vi "PvgeneratorOP300.vi"(8 "errin":errorcluster, 10 "network":path, 11 "path in":path) -> (0 "sortie d'erreur":errorcluster caption="errout", 1 "network out":path, 2 "tout bon":bool, 3 "Chaîne":string)   [LabVIEW 2020]
uses:
  SubVI/CheminDeBase.vi
  VG/IS30%.vi
  VG/PN.vi
  <vilib>/Utility/config.llb/NI_LVConfig.lvlib
panel:
  out "nombre de remplacements":i32
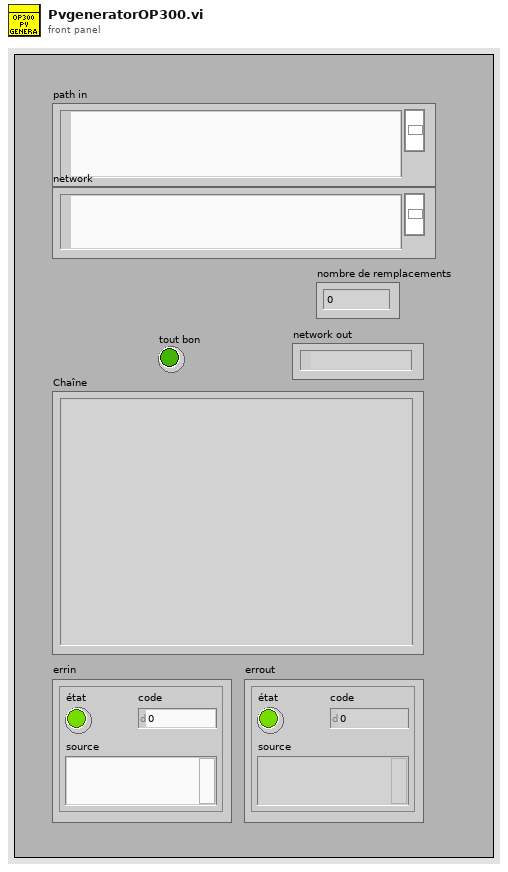
[diagram p1: front panel]
types:
  T1 = enum16{"open", "replace", "create", "open or create", "replace or create", "replace or create with confirmation"}
  T2 = typedef "NI_LVConfig.lvlib/Config Data RefNum.ctl" = refnum<k1>
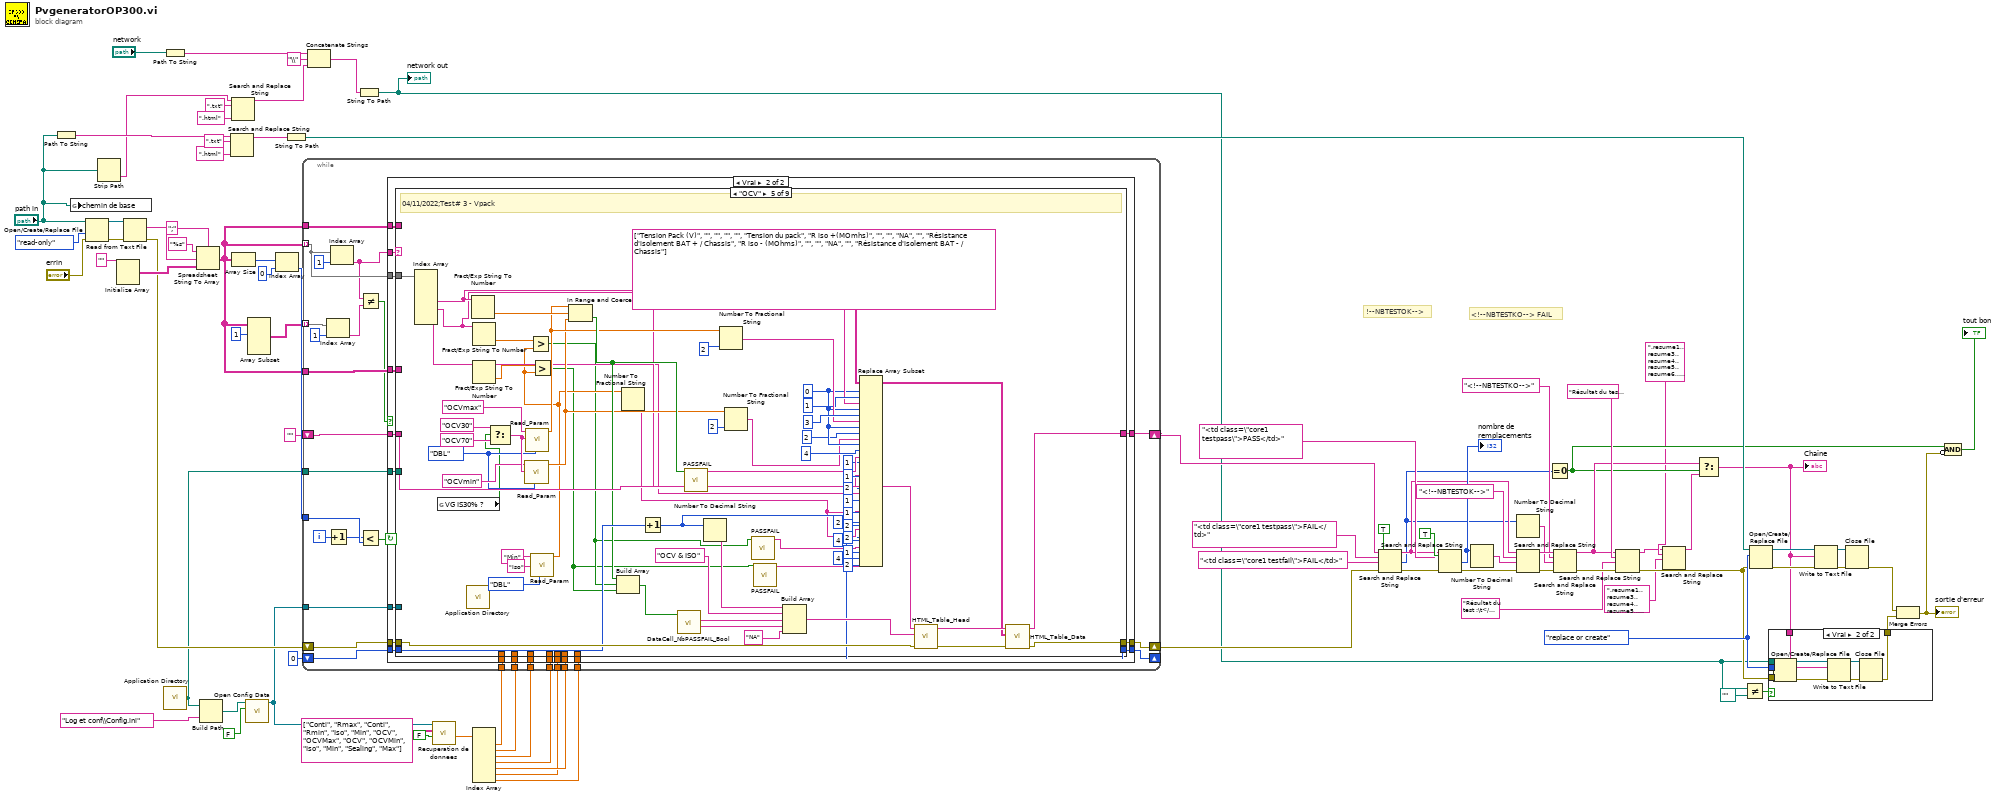
[diagram p0: block diagram]
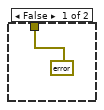
[diagram p2: hidden frame]
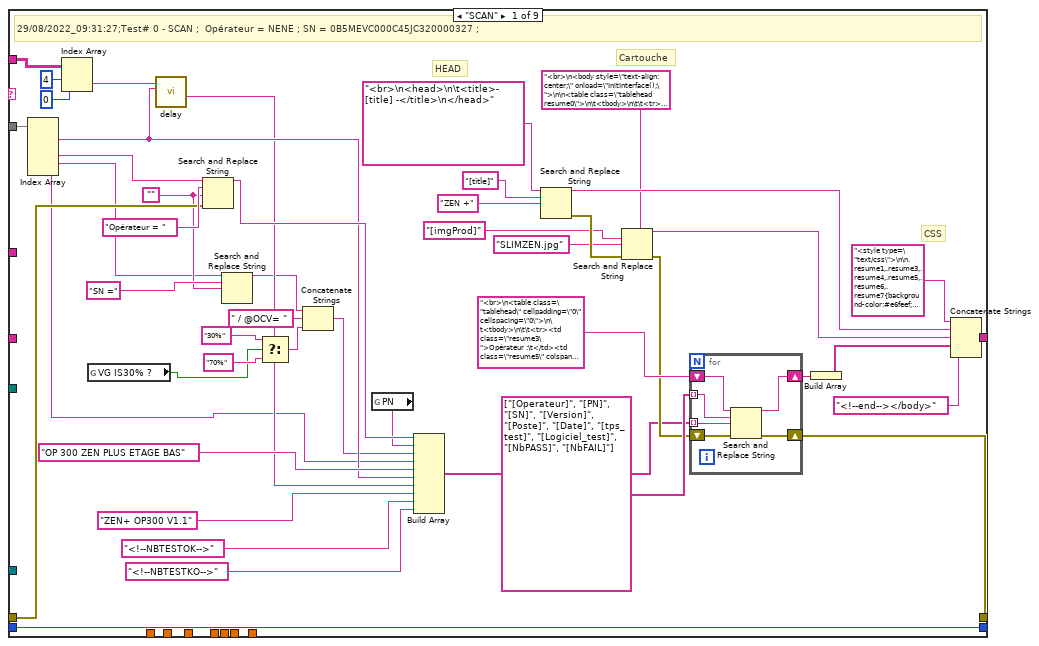
[diagram p4: hidden frame]
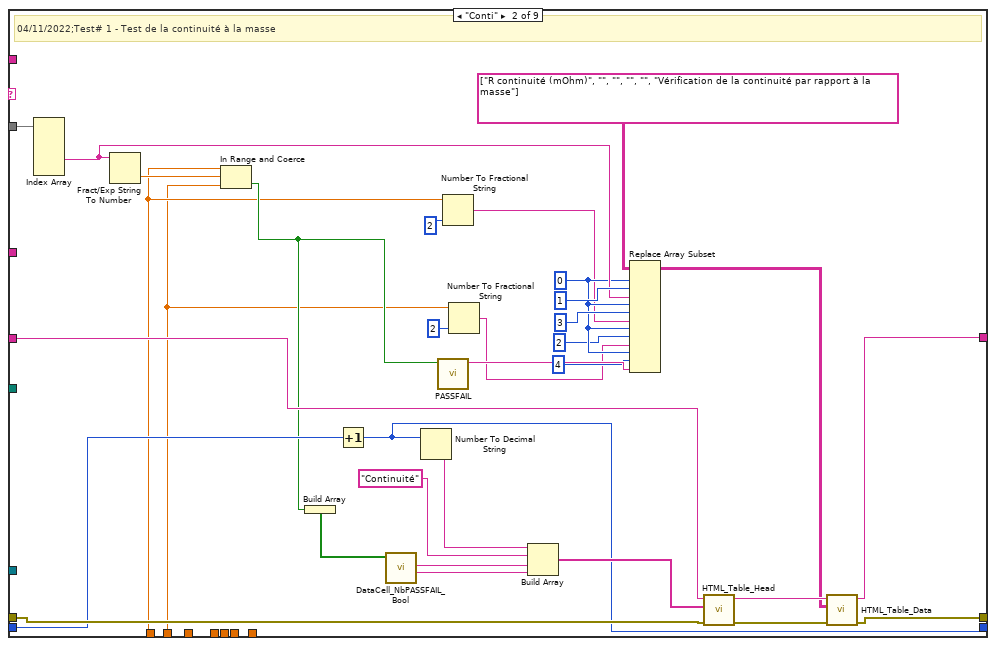
[diagram p5: hidden frame]
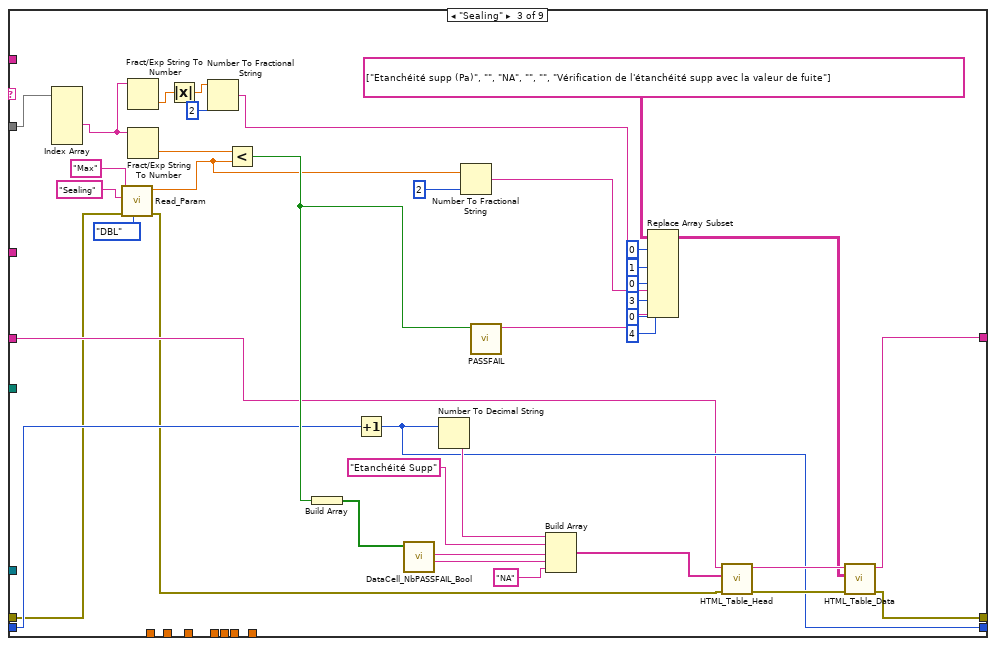
[diagram p6: hidden frame]
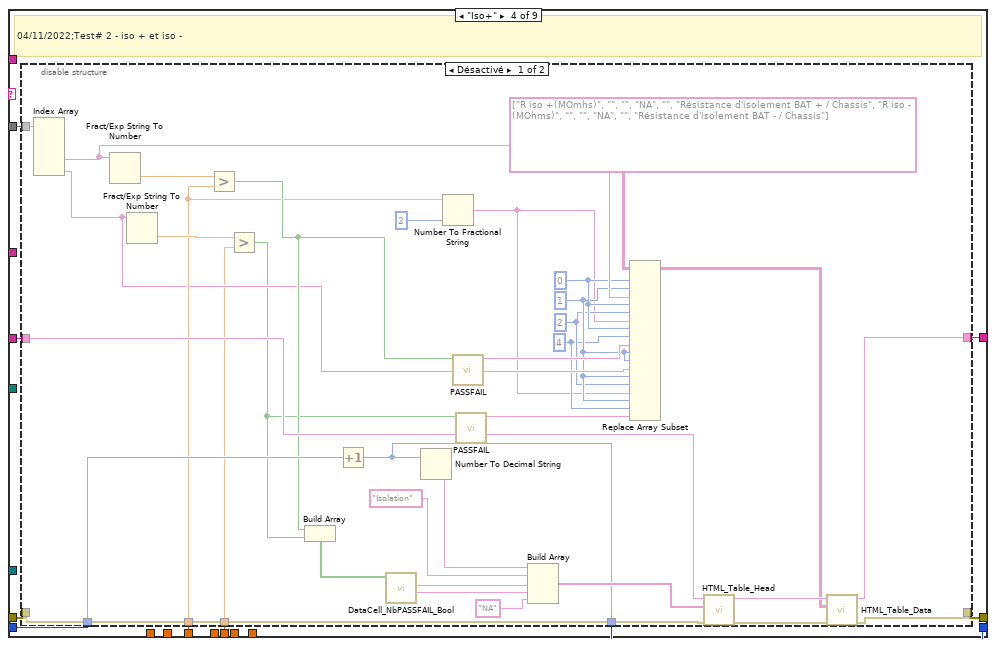
[diagram p7: hidden frame]
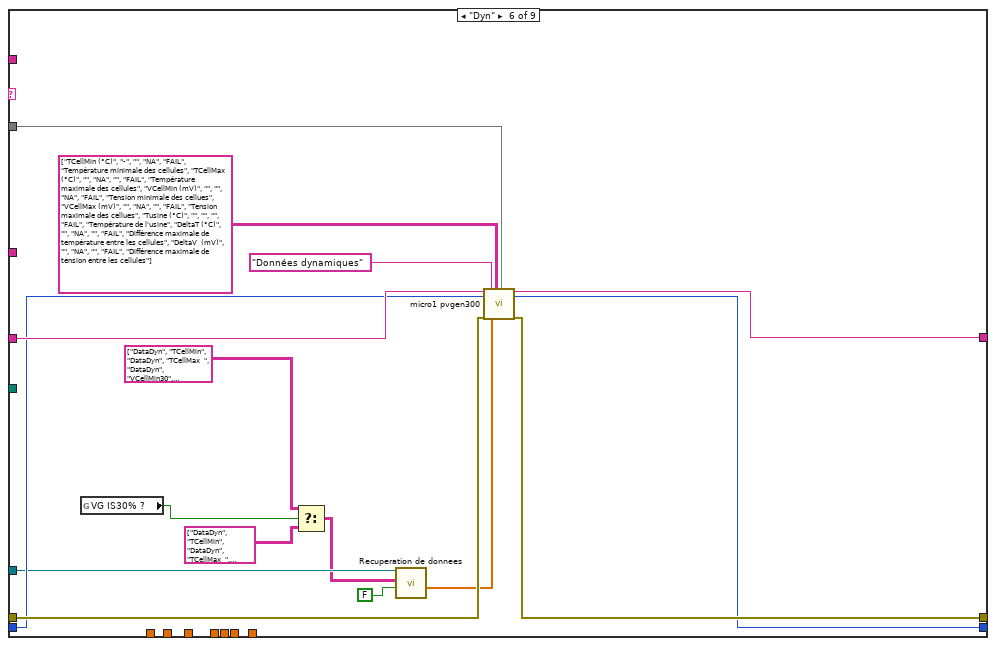
[diagram p9: hidden frame]
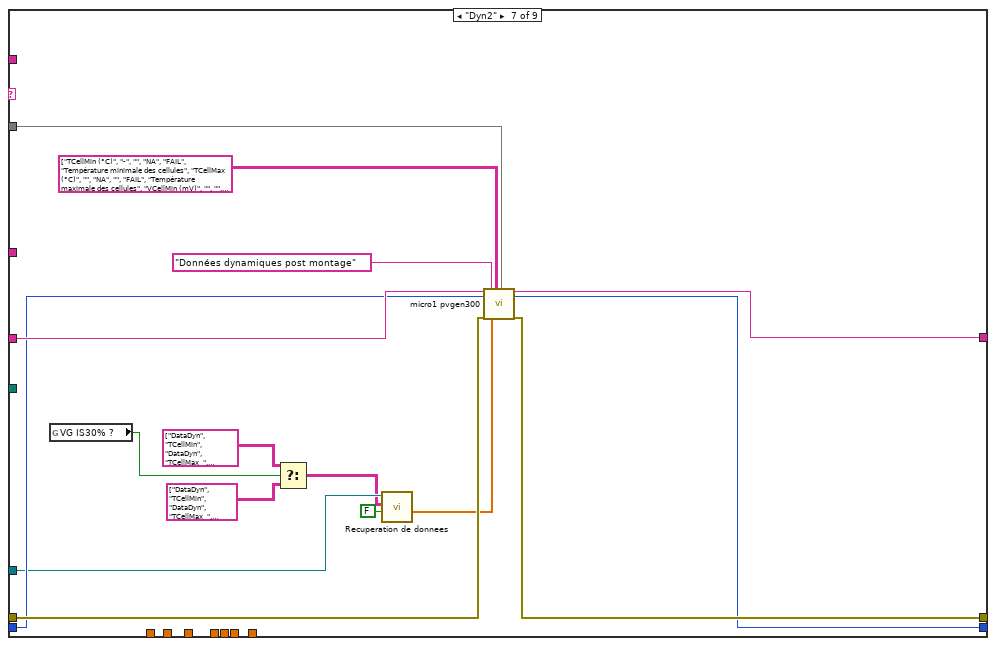
[diagram p10: hidden frame]
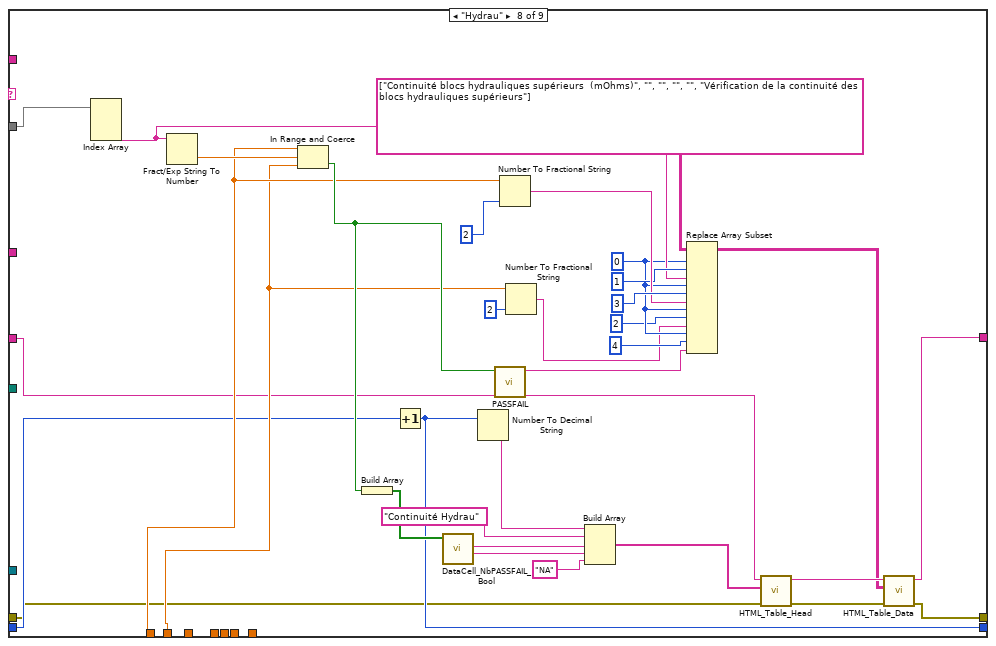
[diagram p11: hidden frame]
diagram:
  w47 = T1."replace or create" ("opération (0 : open)")
  # "<!--NBTESTKO--> FAIL"
  # "!--NBTESTOK-->"
  n1 = Path To String(path="path in") -> (string=w69:string)
  n2 = global write "CheminDeBase.vi" "chemin de base"("path in") -> ()
  n3 = Open/Create/Replace File(file path (use dialog)="path in", error in="errin", access (0:read/write)=enum16{"read/write", "read-only", "write-only"}."read-only" ("accès (0 : read/write)")) -> (refnum out=w70:refnum<file>, error out=w87:errorcluster)  [unwired: 3 in, 1 out]
  n4 = Strip Path(path="path in") -> (name=w29:string)  [unwired: 1 out]
  n5 = Initialize Array("") -> (w85:string[][])  [unwired: 2 in]
  n6 = Read from Text File(file (use dialog)=w70, error in=w87) -> (text=w83:string, error out=w75:errorcluster)  [unwired: 2 in, 2 out]
  n7 = Path To String(path="network") -> (string=w28:string)
  n8 = call <vilib>:"Application Directory.vi"() -> ("Application Directory"=w2:path)
  n9 = Spreadsheet String To Array(delimiter (Tab)=";" ("séparateur (Tabulation)"), format string="%s" ("chaîne de format"), spreadsheet string=w83, array type (2D Dbl)=w85) -> (array=w8:string[][])
  n10 = Build Path(base path=w2, name or relative path="Log et conf\\Config.ini") -> (appended path=w23:path)
  n11 = Search and Replace String(input string=w69, search string=".txt" ("chaîne recherchée"), replace string=".html" ("chaîne de remplacement (\"\")")) -> (result string=w66:string)  [unwired: 5 in, 3 out]
  n12 = Search and Replace String(input string=w29, search string=".txt" ("chaîne recherchée"), replace string=".html" ("chaîne de remplacement (\"\")")) -> (result string=w26:string)  [unwired: 5 in, 3 out]
  n13 = Array Size(array=w8) -> (size(s)=w81:i32[])
  n14 = call <vilib>:"Open Config Data.vi"("create file if necessary (T)"=FALSE, "configuration file path"=w23) -> ("refnum"=w3:T2)  [unwired: 7 in, 2 out]
  n15 = Array Subset(array=w8, index (row)=1 ("indice")) -> (w6:string[][])  [unwired: 3 in]
  n16 = Index Array(array=w81, index=0 ("indice")) -> (element=w79:i32)
  n17 = String To Path(string=w66) -> (path=w65:path)
  n18 = Concatenate Strings(w28, "\\" ("chaîne"), w26) -> (w25:string)
  n19 = String To Path(string=w25) -> (path=w30:path)
  "network out" <- w30
  n20 = call "Recuperation de donnees.vi"("Est-ce un string?"=FALSE, "Array in"=string[][] [["Conti", "Rmax"], ["Conti", "Rmin"], ["Iso", "Min"], ["OCV", "OCVMax"], ["OCV", "OCVMin"], ["Iso", "Min"], ["Sealing", "Max"]], "Refnum in"=w3) -> ("Array"=w18:dbl[])  [unwired: 7 in, 1 out]
  n21 = Index Array(array=w18) -> (element #1=w17:dbl, element #2=w16:dbl, element #3=w15:dbl, element #4=w14:dbl, element #5=w13:dbl, element #6=w5:dbl, element #7=w4:dbl)  [unwired: 7 in]
  n22 = while {
    tunnel: w79 -> [w115]
    tunnel: w8 -> [w112] mode=indexing
    shift-right: [w111] -> w62
    shift-left: w75 -> [w110]
    shift-right: [w104] -> w64
    shift-left: "" -> [w109]
    shift-right: [w107] -> _
    shift-left: 0 -> [w108]
    tunnel: w8 -> [w106]
    tunnel: w17 -> [w103]
    tunnel: w16 -> [w102]
    tunnel: w8 -> [w101]
    tunnel: w15 -> [w100]
    tunnel: w14 -> [w99]
    tunnel: w13 -> [w98]
    tunnel: w6 -> [w96] mode=indexing
    tunnel: w5 -> [w92]
    tunnel: w4 -> [w91]
    tunnel: w3 -> [w90]
    tunnel: w2 -> [w89]
    i -> [w116]
    stop <- w114 continue-if-true
    n23 = Index Array(array=w96, index=1 ("indice")) -> (element=w95:string)
    n24 = Increment(x=w116) -> (x+1=w105:i32)
    n25 = Index Array(array=w112, index=1 ("indice")) -> (element=w94:string)
    n26 = Less?(x=w105, y=w115) -> (x < y?=w114:bool)
    n27 = Not Equal?(x=w94, y=w95) -> (x != y?=w93:bool)
    n28 = case shown="Vrai" w93 {
      tunnel: w112 -> [_ w138]
      tunnel: [w118 w137] -> w111
      tunnel: w110 -> [w118 w136]
      tunnel: w109 -> [w119 w135]
      tunnel: w108 -> [w117 w134]
      tunnel: [w117 w133] -> w107
      tunnel: w106 -> [_ w132]
      tunnel: [w119 w131] -> w104
      tunnel: w94 -> [_ w130]
      tunnel: w103 -> [_ w120]
      tunnel: w102 -> [_ w129]
      tunnel: w101 -> [_ w128]
      tunnel: w100 -> [_ w127]
      tunnel: w99 -> [_ w126]
      tunnel: w98 -> [_ w125]
      tunnel: w92 -> [_ w124]
      tunnel: w91 -> [_ w123]
      tunnel: w90 -> [_ w122]
      tunnel: w89 -> [_ w121]
      frame False {
      }
      frame True {
        n29 = case shown="\"OCV\"" w130 {
          tunnel: w136 -> [w183 w216 w231 w270 w362 w386 w402 w405 w438]
          tunnel: w138 -> [w185 w217 w246 w271 w363 w383 w399 w411 _]
          tunnel: [w162 w215 w235 w269 w361 w385 w401 w406 w438] -> w137
          tunnel: w135 -> [_ w214 w232 w268 w360 w382 w398 w404 w436]
          tunnel: w134 -> [w161 w213 w234 w267 w359 w381 w397 w408 w437]
          tunnel: [w161 w212 w233 w266 w358 w380 w396 w407 w437] -> w133
          tunnel: w132 -> [_ _ _ _ _ _ _ _ _]
          tunnel: [w160 w211 w236 w265 w357 w384 w400 w403 w436] -> w131
          tunnel: w129 -> [_ w194 _ _ _ _ _ w409 _]
          tunnel: w128 -> [w154 _ _ _ _ _ _ _ _]
          tunnel: w127 -> [_ _ _ w264 _ _ _ _ _]
          tunnel: w126 -> [_ _ _ _ _ _ _ _ _]
          tunnel: w125 -> [_ _ _ _ _ _ _ _ _]
          tunnel: w124 -> [_ _ _ w263 _ _ _ _ _]
          tunnel: w123 -> [_ _ _ _ _ _ _ _ _]
          tunnel: w122 -> [_ _ _ _ _ w379 w395 _ _]
          tunnel: w121 -> [_ _ _ _ _ _ _ _ _]
          tunnel: w120 -> [_ w195 _ _ _ _ _ w410 _]
          frame "SCAN" {
            w156 = ""
            # "Cartouche"
            # "HEAD"
            # "CSS"
            # "29/08/2022_09:31:27;Test# 0 - SCAN ;  Opérateur = NENE ; SN = 0B5MEVC000C45JC320000327 ;"
            n30 = Index Array(array=w185) -> (element #1=w150:string, element #3=w159:string, element #4=w155:string, element #5=w139:string)  [unwired: 5 in, 1 out]
            n31 = Index Array(array=w154, index (row)=4, index (col)=0 ("disabled index (col)")) -> (element=w151:string)
            n32 = global read "IS30%.vi" "VG IS30% ?"() -> (w141:bool)
            n33 = call "delay.vi"("String"=w150, "String 2"=w151) -> ("Delay calculé"=w149:string)  [unwired: 9 in]
            n34 = Search and Replace String(input string=w159, search string="Opérateur = " ("chaîne recherchée"), replace string=w156, error in=w183) -> (result string=w158:string)  [unwired: 4 in, 3 out]
            n35 = Search and Replace String(input string=w155, search string="SN =" ("chaîne recherchée"), replace string=w156) -> (result string=w147:string)  [unwired: 5 in, 3 out]
            n36 = Select(t="30%" ("y"), s=w141, f="70%" ("y")) -> (s? t:f=w144:string)
            n37 = Concatenate Strings(w147, " / @OCV= " ("chaîne"), w144) -> (w146:string)
            n38 = global read "PN.vi" "PN"() -> (w140:string)
            n39 = Build Array(w158, w140, w146, w139, "OP 300 ZEN PLUS ETAGE BAS" ("chaîne"), w150, w149, "ZEN+ OP300 V1.1" ("chaîne"), "<!--NBTESTOK-->" ("chaîne"), "<!--NBTESTKO-->" ("chaîne")) -> (w163:string[])
            n40 = Search and Replace String(input string="<br>\n<head>\n\t<title>- [title] -</title>\n</head>", search string="[title]" ("chaîne recherchée"), replace string="ZEN +" ("Title")) -> (result string=w179:string, error out=w178:errorcluster)  [unwired: 5 in, 2 out]
            n41 = Search and Replace String(input string="<br>\n<body style=\"text-align: center;\" onload=\"InitInterface();\">\n\n<table class=\"tablehead resume0\">\n\t<tbody>\n\t\t<tr>\n\t\t\t<td> <img src=\"[imgProd]\" style=\"width:194px;height:100px\" class=\"left\"></td>\n\t\t\t<td> <div class=\"center\">PROCES VERBAL DE TEST AUTOMATIQUE</div><div class=\"center\">Zen Plus OP 300</div><br class=\"center\"><div class=\"center\">Forseepower</div></td>\n\t\t\t<td> <img src=\"LOGO FORSEE.png\" style=\"width:194px;height:100px\"  class=\"right\"></td>\n\t\t</tr>\n\t</tbody>\n</table>", search string="[imgProd]", replace string="SLIMZEN.jpg" ("imgProd"), error in=w178) -> (result string=w176:string, error out=w173:errorcluster)  [unwired: 4 in, 2 out]
            n42 = for {
              shift-right: [w190] -> w172
              shift-left: "<br>\n<table class=\"tablehead\" cellpadding=\"0\" cellspacing=\"0\">\n\t<tbody>\n\t\t<tr><td class=\"resume3\">Opérateur :\t</td><td class=\"resume5\" colspan=\"3\">[Operateur]</td></tr>\n\t\t<tr><td class=\"resume3\">PN : </td><td class=\"resume5\" colspan=\"3\">[PN]</td></tr>\n\t\t<tr><td class=\"resume3\">SN : </td><td class=\"resume5\" colspan=\"3\">[SN]</td></tr>\n\t\t<tr><td class=\"resume3\">Version : </td><td class=\"resume5\" colspan=\"3\">[Version]</td></tr>\n\t\t<tr><td class=\"resume3\">Poste : </td><td class=\"resume5\" colspan=\"3\">[Poste]</td></tr>\t\t\n\t\t<tr><td class=\"resume3\">Date du test : </td><td class=\"resume5\" colspan=\"3\">[Date]</td></tr>\n\t\t<tr><td class=\"resume3\">Temps de test : </td><td class=\"resume5\" colspan=\"3\">[tps_test]</td></tr>\n\t\t<tr><td class=\"resume3\">Logiciel de test :\t</td><td class=\"resume5\" colspan=\"3\">[Logiciel_test]</td></tr>\n\t\t<tr><td class=\"resume3\">Résultat du test :\t</td><td class=\"resume5\" colspan=\"3\"><div><span style=\"float:left\" id=\"result\"><font size = \"5pt\" color=\"green\"><b>CONFORME</b></font><b><font size = \"5pt\"> ( </font><font size = \"5pt\" color=\"green\">[NbPASS] PASS </font>  <font size = \"5pt\"> / </font><font size = \"5pt\" color=\"red\">[NbFAIL] FAIL</font> <font size = \"5pt\"> ) </font></b></span></div></td></tr>\n\t</tbody>\n</table>" -> [w191]
              tunnel: string[] ["[Operateur]", "[PN]", "[SN]", "[Version]", "[Poste]", "[Date]", "[tps_test]", "[Logiciel_test]", "[NbPASS]", "[NbFAIL]"] -> [w187] mode=indexing
              tunnel: w163 -> [w186] mode=indexing
              shift-right: [w188] -> w162
              shift-left: w173 -> [w189]
              n43 = Search and Replace String(input string=w191, search string=w187, replace string=w186, error in=w189) -> (result string=w190:string, error out=w188:errorcluster)  [unwired: 4 in, 2 out]
            }
            n44 = Build Array(w172) -> (w171:string[])
            n45 = Concatenate Strings("<style type=\"text/css\">\n\n.resume1,.resume3,.resume4,.resume5,.resume6,.resume7{background-color:#e6feef;padding:7px;border:1px solid black;}\n.resume0{border:1px solid black;background-color:#e6feef;font-weight: bold;padding:0px;text-align: center;}\n.resume1{width:350px;text-align:right;font-weight:bold;}\n.resume3{width:350px;text-align:right;border-top:0px solid black;font-weight:bold;}\n.resume4{border-left:0px solid black;width:290px;}\n.resume5{width:290px;border-left:0px solid black;border-top:0px solid black;}\n.resume6{border-left:0px solid black;width:60px;}\n.resume7{border-left:0px solid black;border-top:0px solid black;width:60px;}\n.title1{text-align: left;background-color:#e6f4fe;padding:10px;border:1px solid #101010;}\n.title2{width: 30px;text-align: center;background-color:#e6f4fe;padding:1px;border:1px solid #101010;border-left:0px solid black;font-weight: bold;}\n.title2 a:link{text-decoration:none;}\n.entete0,.entete1,.entete2,.time2{text-align: center;background-color:#feeec9;padding:7px;border:1px solid black;font-weight: bold;}\n.entete0{width:45px;border-right:0px solid black;}\n.entete1{width:505px;}\n.entete2{width:95px;border-right:0px solid black;}\n.time2{border-left:0px solid black;width:145px;font-size:11px;}\n.core0,.core1,.core2,.core3,.core4,.time{text-align: center;background-color:#fafed3;padding:7px;border:1px solid black;}\n.core0, .core1,.core3,.core4{width:95px;border-top:0px solid black;border-right:0px solid black;}\n.core0{width:45px;}\n.core2{border-top:0px solid black;width:505px;}\n.core3{width:200px;}\n.core4{width:300px;}\n.time{width:145px;border-top:0px solid black;border-left:0px solid black;font-size:11px;}\n.false .core0,.false .core1,.false .core2,.false .core3,.false .core4,.false .time{background-color:#f4f4f4;}\n.false .entete0,.false .entete1,.false .entete2,.false .time2{background-color:#dadada;}\n.false .title1,.false .title2,.false .resultentete .testpass,.false .resultentete .testfail,.false .resultentete .testtime{background-color:#c5cac9;color: blue;}\n.false .title2 a:link{text-decoration:none;color: blue;}\n.comment1,.comment2,.time3{width: 890px;background-color:#e9e8e9;padding:7px;border:1px solid black;border-top:0px solid black;text-align:left;}\n.comment2{border-right:0px solid black;width: 45px;text-align: center;}\n.time3{width: 145px;border-left:0px solid black;font-size:11px;}\n.fixe1{background: -moz-linear-gradient(center top , #101010 10%, #555555 80%) repeat scroll 0 0 transparent;background: -webkit-gradient(linear, left top, left bottom, from(#101010), to(#555555));border:2px solid orange;position : fixed;margin-top:20px;display:none;overflow-y:scroll;max-height:350px;text-shadow: 0px 0px 0 #333333;text-align:left;font-size:10px;padding:10px;margin-left:-162px;border-radius: 15px 15px 15px 15px;}\n.menufixe, .menufixelock{background: -moz-linear-gradient(center top , #101010 80%, transparent 20%) repeat scroll 0 0 transparent;background: -webkit-gradient(linear, left top, left bottom, from(#101010), color-stop(0.65, #101010), to(transparent)) repeat scroll 0 0 transparent;margin: -52px 0px 0px -9px;width:100%;position:fixed;height:55px;-moz-transition: margin 1s;-webkit-transition: margin 1s;}\n.menufixelock, .menufixe:hover{margin: -9px 0px 0px -9px;}\n.lockmenu, .separation,.separationmenu{text-align:center;background: -moz-linear-gradient(center top , #555555 10%, #111111 80%) repeat scroll 0 0 transparent;background: -webkit-gradient(linear, left top, left bottom, from(#555555), to(#111111));border: 1px solid white;border-radius: 10px 10px 10px 10px;box-shadow: 0 -1px 1px #555555 inset;color: #999999;font-weight: bold;width: 100px;padding: 2px;text-decoration: none;}\n.tablehead{width: 1000px;font-family: Verdana;font-size: 12px;margin-left: auto;margin-right: auto;}\n.tablenull{font-family: Verdana;font-size: 11px;margin-left: auto;margin-right: auto;}\n.separationmenu:hover div{display: inline;}\n.lockmenu:hover, .separation:hover,.separationmenu:hover{border: 1px solid orange;cursor:pointer;}\n.lockmenu:hover{border: 1px solid red;cursor:pointer;}\n.separationright{padding:10px;}\ndiv a:link{text-decoration:none;color:#cbcbcb;}\ndiv a:hover{text-decoration:underline;color:#cbcbcb;}\nspan a:link{text-decoration:none;color:#cbcbcb;}\nspan a:hover{text-decoration:none;color:#cbcbcb;}\n.false{color: blue;}\n.testpass{color: green;font-weight: bold;}\n.testfail{color: red;font-weight: bold;}\n.testtime{color: blue;font-weight: bold;}\n.resultentete{font-weight: bold;font-size: 11px;min-width: 200px;text-align:right;}\n.infohard{border: 1px solid black;background-color: white;text-align: center;width: 16px;height: 16px;border-radius: 5px;font-weight: bold;box-shadow: 0 -1px 2px #555555 inset;}\n.infohard:hover{background-color:#feeec9;cursor:pointer;}\n.footerhard{padding-top:30px;}\n.confighard{font-size:10px;width:110px;}\n.circlemain{margin-left:auto;margin-right:auto;}\n.circletext,.circleform{padding-top: 3px;text-align:center;font-size: 10px;width:200px;}\n.circleform{padding-bottom: 3px;padding-top: 1px;}\n.circle{border: 1px solid black;border-collapse: collapse;border-radius: 15px;box-shadow: 1px 1px 0 #505050;height: 15px;width: 15px;display:inline-block;}\n.bookmarkon, .bookmarkoff{background-color: yellow;border: 1px solid black;border-collapse: collapse;border-radius: 10px 10px 10px 10px;box-shadow: 1px 1px 0 #505050;height: 12px;width: 12px;position: absolute;margin-left:22px;cursor: help;}\n.bookmarkoff{background-color: transparent;border: 1px solid #CECECE;box-shadow: none;cursor: copy;}\n.false .bookmarkoff{background-color: transparent;border: 1px solid #E6E1E1;box-shadow: none;cursor: copy;}\n.bookmarkmaster{height: 15px;margin-right: 12px;width: 60px;}\n.bookmarkmaster:hover .bookmarkprev,.bookmarkmaster:hover .bookmarksuiv{display:block;}\n.bookmarkprev, .bookmarksuiv {cursor: pointer;font-size: 25px;font-weight: bold;margin-top: -10px;position: absolute;display:none;}\n.bookmarkprev{margin-left: 2px;}\n.bookmarksuiv{margin-left: 43px;}\n.plus, .moins{background-color: #F4F4F4;border: 1px solid #848484;border-radius: 20px;color: #848484;font-family: arial;font-size: 16px;font-weight: bold;height: 20px;margin-left: 4px;text-align: center;width: 20px;}\n.moins{font-size: 15px;}\n.plus:hover, .moins:hover{background-color: #DADADA;border: 1px solid black;color: black;cursor:pointer;}\n.backtothetop {position: fixed; right: 50%; margin-right: -555px; bottom: 10px; font-size: 35px; font-weight: bold; border: 1px solid #7D7B91; width: 40px; height: 40px; line-height:52px; text-align: center;border-radius: 8px; opacity: 0.25; background-color: #F5F5F5; color:#7D7B91;}\n.backtothetop:hover {opacity: 1; cursor:pointer;}\n.libversion {font-size: 8px;font-weight: normal;padding-right: 10px;text-align: right;}\n.lockmenu {width: 18px;font-size: 12px;}\n.left {display: block; margin-left: 1px;margin-right: auto;}\n.right {display: block; margin-right: 1px;margin-left: auto;}\n.center {display: block; margin-left: auto;margin-right: auto;}\n\n</style>", w179, w176, w171, "<!--end--></body>") -> (w160:string)
          }
          frame "Conti" {
            w199 = 0 ("index (row)")
            # "04/11/2022;Test# 1 - Test de la continuité à la masse"
            n46 = Index Array(array=w217) -> (element #3=w203:string)  [unwired: 5 in, 4 out]
            n47 = Fract/Exp String To Number(string=w203) -> (number=w202:dbl)  [unwired: 3 in, 1 out]
            n48 = In Range and Coerce(upper limit=w195, x=w202, lower limit=w194) -> (In Range?=w197:bool)  [unwired: 1 out]
            n49 = Build Array(w197) -> (w209:bool[])
            n50 = Increment(x=w213) -> (x+1=w212:i32)
            n51 = call <vilib>:"DataCell_NbPASSFAIL_Bool.vi"("Tableau en entrée"=w209) -> ("Chaîne"=w207:string, "Chaîne 2"=w208:string)  [unwired: 8 in, 1 out]
            n52 = Number To Decimal String(number=w212) -> (decimal integer string=w219:string)  [unwired: 1 in]
            n53 = call <vilib>:"PASSFAIL.vi"("E"=w197) -> ("S"=w201:string)  [unwired: 10 in]
            n54 = Number To Fractional String(number=w195, precision (6)=i16 2) -> (F-format string=w192:string)  [unwired: 2 in]
            n55 = Number To Fractional String(number=w194, precision (6)=i16 2) -> (F-format string=w193:string)  [unwired: 2 in]
            n56 = Build Array(w219, "Continuité" ("élément"), w208, w207) -> (w222:string[])
            n57 = Replace Array Subset(array=string[][] [["R continuité (mOhm)", "", "", "", "", "Vérification de la continuité par rapport à la masse"]] ("Tableau"), new element #1=w203, index (row) #1=w199, index (col) #1=1 ("disabled index (col)"), new element #2=w192, index (row) #2=w199, index (col) #2=3 ("disabled index (col)"), new element #3=w193, index (row) #3=w199, index (col) #3=2 ("disabled index (col)"), new element #4=w201, index (row) #4=w199, index (col) #4=4 ("disabled index (col)")) -> (w210:string[][])
            n58 = call "HTML_Table_Head.vi"("entrée d'erreur (pas d'erreur)"=w216, "Tableau"=w222, "chaîne en entrée"=w214) -> ("sortie d'erreur"=w221:errorcluster, "result string"=w220:string)  [unwired: 7 in]
            n59 = call "HTML_Table_Data.vi"("entrée d'erreur (pas d'erreur)"=w221, "Tableau"=w210, "chaîne en entrée"=w220) -> ("sortie d'erreur"=w215:errorcluster, "result string"=w211:string)  [unwired: 7 in]
          }
          frame "Sealing" {
            n60 = Index Array(array=w246) -> (element #3=w228:string)  [unwired: 5 in, 4 out]
            n61 = call "Read_Param.vi"("Énum"=enum16{"STR", "DBL", "U32", "chemin"}."DBL", "errin"=w231, "section"="Sealing", "key"="Max") -> ("error out"=w230:errorcluster, "dbl"=w243:dbl)  [unwired: 3 in, 3 out]
            n62 = Fract/Exp String To Number(string=w228) -> (number=w227:dbl)  [unwired: 3 in, 1 out]
            n63 = Fract/Exp String To Number(string=w228) -> (number=w250:dbl)  [unwired: 3 in, 1 out]
            n64 = Absolute Value(x=w227) -> (abs(x)=w226:dbl)
            n65 = Number To Fractional String(number=w226, precision (6)=i16 2 ("précision (6)")) -> (F-format string=w225:string)  [unwired: 2 in]
            n66 = Less?(x=w250, y=w243) -> (x < y?=w249:bool)
            n67 = Build Array(w249) -> (w254:bool[])
            n68 = Increment(x=w234) -> (x+1=w233:i32)
            n69 = call <vilib>:"DataCell_NbPASSFAIL_Bool.vi"("Tableau en entrée"=w254) -> ("Chaîne"=w252:string, "Chaîne 2"=w253:string)  [unwired: 8 in, 1 out]
            n70 = Number To Decimal String(number=w233) -> (decimal integer string=w258:string)  [unwired: 1 in]
            n71 = Number To Fractional String(number=w243, precision (6)=i16 2) -> (F-format string=w247:string)  [unwired: 2 in]
            n72 = call <vilib>:"PASSFAIL.vi"("E"=w249) -> ("S"=w248:string)  [unwired: 10 in]
            n73 = Build Array(w258, "Etanchéité Supp" ("élément"), w253, w252, "NA" ("élément")) -> (w261:string[])
            n74 = Replace Array Subset(array=string[][] [["Etanchéité supp (Pa)", "", "NA", "", "", "Vérification de l'étanchéité supp avec la valeur de fuite"]] ("Tableau"), new element #1=w225, index (row) #1=0 ("indice (ligne)"), index (col) #1=1 ("indice désactivé (col)"), new element #2=w247, index (row) #2=0 ("indice (ligne)"), index (col) #2=3 ("indice désactivé (col)"), new element #3=w248, index (row) #3=0 ("indice (ligne)"), index (col) #3=4 ("indice désactivé (col)")) -> (w255:string[][])
            n75 = call "HTML_Table_Head.vi"("entrée d'erreur (pas d'erreur)"=w230, "Tableau"=w261, "chaîne en entrée"=w232) -> ("sortie d'erreur"=w260:errorcluster, "result string"=w259:string)  [unwired: 7 in]
            n76 = call "HTML_Table_Data.vi"("entrée d'erreur (pas d'erreur)"=w260, "Tableau"=w255, "chaîne en entrée"=w259) -> ("sortie d'erreur"=w235:errorcluster, "result string"=w236:string)  [unwired: 7 in]
          }
          frame "Iso+" {
            # "04/11/2022;Test# 2 - iso + et iso -"
            n77 = disable-structure shown="Désactivé" {
              disable-tunnel: w271 -> [w298 _]
              disable-tunnel: w270 -> [w297 _]
              disable-tunnel: [w296 _] -> w269
              disable-tunnel: w268 -> [w295 _]
              disable-tunnel: w267 -> [w294 _]
              disable-tunnel: [w293 _] -> w266
              disable-tunnel: [w292 _] -> w265
              disable-tunnel: w264 -> [w281 _]
              disable-tunnel: w263 -> [w272 _]
              frame Disabled {
                w276 = 4 ("disabled index (col)")
                w277 = 2 ("disabled index (col)")
                w278 = 1 ("disabled index (col)")
                w285 = 0 ("index (row)")
                n78 = Index Array(array=w298) -> (element #3=w286:string, element #5=w279:string)  [unwired: 5 in, 3 out]
                n79 = Fract/Exp String To Number(string=w286) -> (number=w284:dbl)  [unwired: 3 in, 1 out]
                n80 = Fract/Exp String To Number(string=w279) -> (number=w282:dbl)  [unwired: 3 in, 1 out]
                n81 = Greater?(x=w284, y=w281) -> (0:w283:bool)
                n82 = Greater?(x=w282, y=w272) -> (0:w274:bool)
                n83 = Build Array(w283, w274) -> (w290:bool[])
                n84 = Increment(x=w294) -> (x+1=w293:i32)
                n85 = call <vilib>:"DataCell_NbPASSFAIL_Bool.vi"("Tableau en entrée"=w290) -> ("Chaîne"=w288:string, "Chaîne 2"=w289:string)  [unwired: 8 in, 1 out]
                n86 = Number To Decimal String(number=w293) -> (decimal integer string=w301:string)  [unwired: 1 in]
                n87 = Number To Fractional String(number=w281, precision (6)=i16 2) -> (F-format string=w275:string)  [unwired: 2 in]
                n88 = call <vilib>:"PASSFAIL.vi"("E"=w283) -> ("S"=w280:string)  [unwired: 10 in]
                n89 = call <vilib>:"PASSFAIL.vi"("E"=w274) -> ("S"=w273:string)  [unwired: 10 in]
                n90 = Build Array(w301, "Isolation" ("élément"), w289, w288, "NA" ("élément")) -> (w304:string[])
                n91 = Replace Array Subset(array=string[][] [["R iso +(MOmhs)", "", "", "NA", "", "Résistance d'isolement BAT + / Chassis"], ["R iso - (MOhms)", "", "", "NA", "", "Résistance d'isolement BAT - / Chassis"]] ("Tableau"), new element #1=w286, index (row) #1=w285, index (col) #1=w278, new element #2=w275, index (row) #2=w285, index (col) #2=w277, new element #3=w280, index (row) #3=w285, index (col) #3=w276, new element #4=w279, index (row) #4=w278, index (col) #4=w278, new element #5=w275, index (row) #5=w278, index (col) #5=w277, new element #6=w273, index (row) #6=w278, index (col) #6=w276) -> (w291:string[][])
                n92 = call "HTML_Table_Head.vi"("entrée d'erreur (pas d'erreur)"=w297, "Tableau"=w304, "chaîne en entrée"=w295) -> ("sortie d'erreur"=w303:errorcluster, "result string"=w302:string)  [unwired: 7 in]
                n93 = call "HTML_Table_Data.vi"("entrée d'erreur (pas d'erreur)"=w303, "Tableau"=w291, "chaîne en entrée"=w302) -> ("sortie d'erreur"=w296:errorcluster, "result string"=w292:string)  [unwired: 7 in]
              }
              frame Enabled {
              }
            }
          }
          frame "OCV" {
            w334 = enum16{"STR", "DBL", "U32"}."DBL" ("Énum")
            w344 = 0 ("index (row)")
            # "04/11/2022;Test# 3 - Vpack"
            n94 = Index Array(array=w363) -> (element #3=w348:string, element #5=w324:string, element #7=w321:string)  [unwired: 7 in, 4 out]
            n95 = global read "IS30%.vi" "VG IS30% ?"() -> (w331:bool)
            n96 = call <vilib>:"Application Directory.vi"() -> ()  [unwired: 1 out]
            n97 = Fract/Exp String To Number(string=w348) -> (number=w347:dbl)  [unwired: 3 in, 1 out]
            n98 = Fract/Exp String To Number(string=w324) -> (number=w330:dbl)  [unwired: 3 in, 1 out]
            n99 = Fract/Exp String To Number(string=w321) -> (number=w327:dbl)  [unwired: 3 in, 1 out]
            n100 = Select(t="OCV30" ("section"), s=w331, f="OCV70" ("section")) -> (s? t:f=w337:string)
            n101 = call "Read_Param.vi"("Énum"=w334, "section"=w337, "key"="OCVmin") -> ("dbl"=w332:dbl)  [unwired: 4 in, 4 out]
            n102 = call "Read_Param.vi"("Énum"=w334, "section"=w337, "key"="OCVmax") -> ("dbl"=w333:dbl)  [unwired: 4 in, 4 out]
            n103 = call "Read_Param.vi"("Énum"=enum16{"STR", "DBL", "U32", "chemin"}."DBL", "section"="Iso", "key"="Min") -> ("dbl"=w320:dbl)  [unwired: 4 in, 4 out]
            n104 = Greater?(x=w330, y=w320) -> (0:w314:bool)
            n105 = Greater?(x=w327, y=w320) -> (0:w313:bool)
            n106 = In Range and Coerce(upper limit=w333, x=w347, lower limit=w332) -> (In Range?=w342:bool)  [unwired: 1 out]
            n107 = Build Array(w342, w314, w313) -> (w355:bool[])
            n108 = Number To Fractional String(number=w320) -> (F-format string=w317:string)  [unwired: 3 in]
            n109 = Increment(x=w359) -> (x+1=w358:i32)
            n110 = call <vilib>:"DataCell_NbPASSFAIL_Bool.vi"("Tableau en entrée"=w355) -> ("Chaîne"=w353:string, "Chaîne 2"=w354:string)  [unwired: 8 in, 1 out]
            n111 = call <vilib>:"PASSFAIL.vi"("E"=w342) -> ("S"=w346:string)  [unwired: 10 in]
            n112 = Number To Decimal String(number=w358) -> (decimal integer string=w366:string)  [unwired: 1 in]
            n113 = Number To Fractional String(number=w333, precision (6)=i16 2) -> (F-format string=w351:string)  [unwired: 2 in]
            n114 = Number To Fractional String(number=w332, precision (6)=i16 2) -> (F-format string=w340:string)  [unwired: 2 in]
            n115 = call <vilib>:"PASSFAIL.vi"("E"=w314) -> ("S"=w312:string)  [unwired: 10 in]
            n116 = call <vilib>:"PASSFAIL.vi"("E"=w313) -> ("S"=w309:string)  [unwired: 10 in]
            n117 = Build Array(w366, "OCV & ISO" ("élément"), w354, w353, "NA" ("élément")) -> (w369:string[])
            n118 = Replace Array Subset(array=string[][] [["Tension Pack (V)", "", "", "", "", "Tension du pack"], ["R iso +(MOmhs)", "", "", "NA", "", "Résistance d'isolement BAT + / Chassis"], ["R iso - (MOhms)", "", "", "NA", "", "Résistance d'isolement BAT - / Chassis"]] ("Tableau"), new element #1=w348, index (row) #1=w344, index (col) #1=1 ("disabled index (col)"), new element #2=w351, index (row) #2=w344, index (col) #2=3 ("disabled index (col)"), new element #3=w340, index (row) #3=w344, index (col) #3=2 ("disabled index (col)"), new element #4=w346, index (row) #4=w344, index (col) #4=4 ("disabled index (col)"), new element #5=w324, index (row) #5=1 ("indice (ligne)"), index (col) #5=1 ("indice désactivé (col)"), new element #6=w321, index (row) #6=2 ("indice (ligne)"), index (col) #6=1 ("indice désactivé (col)"), new element #7=w317, index (row) #7=1 ("indice (ligne)"), index (col) #7=2 ("indice désactivé (col)"), new element #8=w317, index (row) #8=2 ("indice (ligne)"), index (col) #8=2 ("indice désactivé (col)"), new element #9=w312, index (row) #9=1 ("indice (ligne)"), index (col) #9=4 ("indice désactivé (col)"), new element #10=w309, index (row) #10=2 ("indice (ligne)"), index (col) #10=4 ("indice désactivé (col)")) -> (w356:string[][])
            n119 = call "HTML_Table_Head.vi"("entrée d'erreur (pas d'erreur)"=w362, "Tableau"=w369, "chaîne en entrée"=w360) -> ("sortie d'erreur"=w368:errorcluster, "result string"=w367:string)  [unwired: 7 in]
            n120 = call "HTML_Table_Data.vi"("entrée d'erreur (pas d'erreur)"=w368, "Tableau"=w356, "chaîne en entrée"=w367) -> ("sortie d'erreur"=w361:errorcluster, "result string"=w357:string)  [unwired: 7 in]
          }
          frame "Dyn" {
            n121 = global read "IS30%.vi" "VG IS30% ?"() -> (w372:bool)
            n122 = Select(t=string[][] [["DataDyn", "TCellMin"], ["DataDyn", "TCellMax  "], ["DataDyn", "VCellMin30"], ["DataDyn", "VCellMax30"], ["DataDyn", "TusineMax"], ["DataDyn", "TusineMin"], ["DataDyn", "DeltaT "], ["DataDyn", "DeltaV "]], s=w372, f=string[][] [["DataDyn", "TCellMin"], ["DataDyn", "TCellMax  "], ["DataDyn", "VCellMin70 "], ["DataDyn", "VCellMax70"], ["DataDyn", "TusineMax"], ["DataDyn", "TusineMin"], ["DataDyn", "DeltaT "], ["DataDyn", "DeltaV "]]) -> (s? t:f=w373:string[][])
            n123 = call "Recuperation de donnees.vi"("Est-ce un string?"=FALSE, "Array in"=w373, "Refnum in"=w379) -> ("Array"=w375:dbl[])  [unwired: 7 in, 1 out]
            n124 = call "micro1 pvgen300.vi"("FluxStrIn"=w382, "Numin"=w381, "errin"=w386, "testlabel"="Données dynamiques", "Data limit"=w375, "tab ref"=string[][] [["TCellMin (°C)", "-", "", "NA", "FAIL", "Température minimale des cellules"], ["TCellMax (°C)", "", "NA", "", "FAIL", "Température maximale des cellules"], ["VCellMin (mV)", "", "", "NA", "FAIL", "Tension minimale des cellues"], ["VCellMax (mV)", "", "NA", "", "FAIL", "Tension maximale des cellues"], ["Tusine (°C)", "", "", "", "FAIL", "Température de l'usine"], ["DeltaT (°C)", "", "NA", "", "FAIL", "Différence maximale de température entre les cellules"], ["DeltaV  (mV)", "", "NA", "", "FAIL", "Différence maximale de tension entre les cellules"]] ("Tableau"), "ligne à traiter"=w383) -> ("result string"=w384:string, "Numout"=w380:i32, "errout"=w385:errorcluster)  [unwired: 10 in]
          }
          frame "Dyn2" {
            n125 = global read "IS30%.vi" "VG IS30% ?"() -> (w387:bool)
            n126 = Select(t=string[][] [["DataDyn", "TCellMin"], ["DataDyn", "TCellMax  "], ["DataDyn", "VCellMin30"], ["DataDyn", "VCellMax30"], ["DataDyn", "TusineMax"], ["DataDyn", "TusineMin"], ["DataDyn", "DeltaT "], ["DataDyn", "DeltaV "]], s=w387, f=string[][] [["DataDyn", "TCellMin"], ["DataDyn", "TCellMax  "], ["DataDyn", "VCellMin70 "], ["DataDyn", "VCellMax70"], ["DataDyn", "TusineMax"], ["DataDyn", "TusineMin"], ["DataDyn", "DeltaT "], ["DataDyn", "DeltaV "]]) -> (s? t:f=w389:string[][])
            n127 = call "Recuperation de donnees.vi"("Est-ce un string?"=FALSE, "Array in"=w389, "Refnum in"=w395) -> ("Array"=w388:dbl[])  [unwired: 7 in, 1 out]
            n128 = call "micro1 pvgen300.vi"("FluxStrIn"=w398, "Numin"=w397, "errin"=w402, "testlabel"="Données dynamiques post montage", "Data limit"=w388, "tab ref"=string[][] [["TCellMin (°C)", "-", "", "NA", "FAIL", "Température minimale des cellules"], ["TCellMax (°C)", "", "NA", "", "FAIL", "Température maximale des cellules"], ["VCellMin (mV)", "", "", "NA", "FAIL", "Tension minimale des cellues"], ["VCellMax (mV)", "", "NA", "", "FAIL", "Tension maximale des cellues"], ["Tusine (°C)", "", "", "", "FAIL", "Température de l'usine"], ["DeltaT (°C)", "", "NA", "", "FAIL", "Différence maximale de température entre les cellules"], ["DeltaV  (mV)", "", "NA", "", "FAIL", "Différence maximale de tension entre les cellules"]] ("Tableau"), "ligne à traiter"=w399) -> ("result string"=w400:string, "Numout"=w396:i32, "errout"=w401:errorcluster)  [unwired: 10 in]
          }
          frame "Hydrau" {
            w416 = 0 ("index (row)")
            n129 = Index Array(array=w411) -> (element #3=w420:string)  [unwired: 3 in, 2 out]
            n130 = Fract/Exp String To Number(string=w420) -> (number=w419:dbl)  [unwired: 3 in, 1 out]
            n131 = In Range and Coerce(upper limit=w410, x=w419, lower limit=w409) -> (In Range?=w414:bool)  [unwired: 1 out]
            n132 = Build Array(w414) -> (w427:bool[])
            n133 = Increment(x=w408) -> (x+1=w407:i32)
            n134 = call <vilib>:"DataCell_NbPASSFAIL_Bool.vi"("Tableau en entrée"=w427) -> ("Chaîne"=w425:string, "Chaîne 2"=w426:string)  [unwired: 8 in, 1 out]
            n135 = Number To Decimal String(number=w407) -> (decimal integer string=w431:string)  [unwired: 1 in]
            n136 = call <vilib>:"PASSFAIL.vi"("E"=w414) -> ("S"=w418:string)  [unwired: 10 in]
            n137 = Number To Fractional String(number=w410, precision (6)=i16 2) -> (F-format string=w423:string)  [unwired: 2 in]
            n138 = Number To Fractional String(number=w409, precision (6)=i16 2) -> (F-format string=w412:string)  [unwired: 2 in]
            n139 = Build Array(w431, "Continuité Hydrau" ("élément"), w426, w425, "NA" ("élément")) -> (w434:string[])
            n140 = Replace Array Subset(array=string[][] [["Continuité blocs hydrauliques supérieurs  (mOhms)", "", "", "", "", "Vérification de la continuité des blocs hydrauliques supérieurs"]] ("Tableau"), new element #1=w420, index (row) #1=w416, index (col) #1=1 ("disabled index (col)"), new element #2=w423, index (row) #2=w416, index (col) #2=3 ("disabled index (col)"), new element #3=w412, index (row) #3=w416, index (col) #3=2 ("disabled index (col)"), new element #4=w418, index (row) #4=w416, index (col) #4=4 ("disabled index (col)")) -> (w428:string[][])
            n141 = call "HTML_Table_Head.vi"("entrée d'erreur (pas d'erreur)"=w405, "Tableau"=w434, "chaîne en entrée"=w404) -> ("sortie d'erreur"=w433:errorcluster, "result string"=w432:string)  [unwired: 7 in]
            n142 = call "HTML_Table_Data.vi"("entrée d'erreur (pas d'erreur)"=w433, "Tableau"=w428, "chaîne en entrée"=w432) -> ("sortie d'erreur"=w406:errorcluster, "result string"=w403:string)  [unwired: 7 in]
          }
          frame "NULL", Default {
            # "NULL"
          }
        }
      }
    }
  }
  n143 = Search and Replace String(replace all?=TRUE ("tout remplacer ? (F)"), input string=w64, search string="<td class=\"core1 testpass\">FAIL</td>" ("chaîne recherchée"), replace string="<td class=\"core1 testfail\">FAIL</td>" ("chaîne de remplacement (\"\")"), error in=w62) -> (result string=w48:string, number of replacements=w43:i32, error out=w59:errorcluster)  [unwired: 3 in, 1 out]
  n144 = Search and Replace String(replace all?=TRUE ("tout remplacer ? (F)"), input string=w48, search string="<td class=\"core1 testpass\">PASS</td>" ("chaîne recherchée"), error in=w59) -> (number of replacements=w51:i32, error out=w55:errorcluster)  [unwired: 4 in, 2 out]
  "nombre de remplacements" <- w51
  n145 = Number To Decimal String(number=w51) -> (decimal integer string=w50:string)  [unwired: 1 in]
  n146 = Number To Decimal String(number=w43) -> (decimal integer string=w49:string)  [unwired: 1 in]
  n147 = Search and Replace String(input string=w48, search string="<!--NBTESTOK-->" ("chaîne recherchée"), replace string=w50, error in=w55) -> (result string=w56:string, error out=w54:errorcluster)  [unwired: 4 in, 2 out]
  n148 = Equal To 0?(x=w43) -> (x = 0?=w35:bool)
  n149 = Search and Replace String(input string=w56, search string="<!--NBTESTKO-->" ("chaîne recherchée"), replace string=w49, error in=w54) -> (result string=w38:string, error out=w42:errorcluster)  [unwired: 4 in, 2 out]
  n150 = Search and Replace String(input string=w38, search string="Résultat du test :\t</td><td class=\"resume5\" colspan=\"3\"><div><span style=\"float:left\" id=\"result\"><font size = \"5pt\" color=\"green\"><b>CONFORME</b>", replace string="Résultat du test :\t</td><td class=\"resume5\" colspan=\"3\"><div><span style=\"float:left\" id=\"result\"><font  size = \"5pt\" color=\"red\"><b>NON CONFORME</b>", error in=w42) -> (result string=w10:string, error out=w41:errorcluster)  [unwired: 4 in, 2 out]
  n151 = Search and Replace String(input string=w10, search string=".resume1,.resume3,.resume4,.resume5,.resume6,.resume7{background-color:#e6feef;padding:7px;border:1px solid black;}\n.resume0{border:1px solid black;background-color:#e6feef;font-weight: bold;padding:0px;text-align: center;}", replace string=".resume1,.resume3,.resume4,.resume5,.resume6,.resume7{background-color:#fdebd0;padding:7px;border:1px solid black;}\n.resume0{border:1px solid black;background-color:#fdebd0;font-weight: bold;padding:0px;text-align: center;}") -> (result string=w9:string)  [unwired: 5 in, 3 out]
  n152 = Select(t=w38, s=w35, f=w9) -> (s? t:f=w39:string)
  "Chaîne" <- w39
  n153 = Not Equal?(x=w30, y=path "") -> (x != y?=w32:bool)
  n154 = Open/Create/Replace File(file path (use dialog)=w65, error in=w41, operation (0:open)=w47) -> (refnum out=w71:refnum<file>, error out=w73:errorcluster)  [unwired: 3 in, 1 out]
  n155 = case shown="Vrai" w32 {
    tunnel: w47 -> [_ w444]
    tunnel: w30 -> [_ w443]
    tunnel: w41 -> [_ w442]
    tunnel: w39 -> [_ w441]
    tunnel: [errorcluster {"status"=FALSE, "code"=0, "source"=""} ("error out") w440] -> w37
    frame False {
    }
    frame True {
      n156 = Open/Create/Replace File(file path (use dialog)=w443, error in=w442, operation (0:open)=w444) -> (refnum out=w445:refnum<file>, error out=w447:errorcluster)  [unwired: 3 in, 1 out]
      n157 = Write to Text File(file (use dialog)=w445, text=w441, error in=w447) -> (refnum out=w446:refnum<file>, error out=w448:errorcluster)  [unwired: 1 in, 1 out]
      n158 = Close File(refnum=w446, error in=w448) -> (error out=w440:errorcluster)  [unwired: 1 out]
    }
  }
  n159 = Write to Text File(file (use dialog)=w71, text=w39, error in=w73) -> (refnum out=w72:refnum<file>, error out=w74:errorcluster)  [unwired: 1 in, 1 out]
  n160 = Close File(refnum=w72, error in=w74) -> (error out=w36:errorcluster)  [unwired: 1 out]
  n161 = Merge Errors(w36, w37) -> (w34:errorcluster)
  "sortie d'erreur" <- w34
  n162 = Compound Arithmetic op=AND ("Opérateur arithmétique")(w35, invert w34) -> (→"tout bon":bool)
